vi "VI Tree - boolean.vi"   [LabVIEW 2020]
uses:
  openg_boolean.lvlib
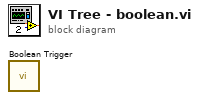
[diagram p0: block diagram]
diagram:
  n1 = call "Boolean Trigger.vi"() -> ()  [unwired: 2 in, 2 out]
